vi "TestStr.vi"() -> ()   [LabVIEW 2025]
uses:
  TestStr.dll
panel:
  out "Get Char from Handle, µs":dbl format="%#.6f"
  out "byte s":u8 format="%.0x"
  out "byte h":u8 format="%.0x"
  out "Ratio":dbl
  out "Get Char from String, s":dbl format="%#_6f"
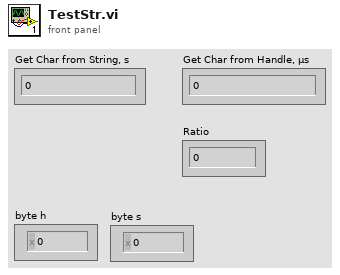
[diagram p1: front panel]
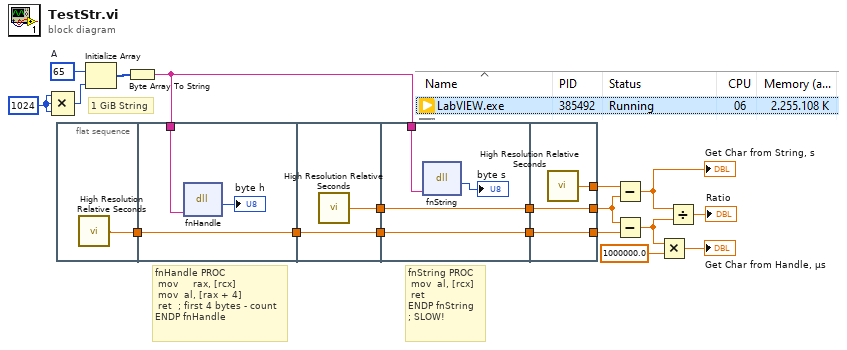
[diagram p0: block diagram]
diagram:
  w17 = 1024
  w19 = u8 65  # A
  # "1 GiB String"
  # "fnString PROC\n\tmov\t\tal, [rcx]\n\tret\nENDP fnString\n; SLOW!"
  # "fnHandle PROC\n\tmov     rax, [rcx]\n\tmov\t\tal, [rax + 4]\n\tret  ; first 4 bytes - count\nENDP fnHandle"
  n1 = Compound Arithmetic op=MULTIPLY(w17, w17, w17) -> (w16:i32)
  n2 = flat-sequence {
    tunnel: [w20] -> w6
    tunnel: w15 -> [w22]
    tunnel: [w23] -> w7
    tunnel: w6 -> [w23]
    tunnel: [w25] -> w13
    tunnel: [w24] -> w8
    tunnel: w7 -> [w24]
    tunnel: w15 -> [w27]
    tunnel: w13 -> [w29]
    tunnel: [w29] -> w12
    tunnel: [w28] -> w9
    tunnel: w8 -> [w28]
    tunnel: [w32] -> w14
    tunnel: w12 -> [w31]
    tunnel: [w31] -> w11
    tunnel: [w30] -> w10
    tunnel: w9 -> [w30]
    frame #0 {
      n3 = call <vilib>:"High Resolution Relative Seconds.vi"() -> ("relative seconds"=w20:dbl)
    }
    frame #1 {
      n4 = dll-call lib="C:/Users/Andrey/Desktop/SlowString&Search/SlowStringIssue/TestStr.dll" fn="fnHandle"("str"=w22) -> ("return type"=→"byte h":u8)  [unwired: 4 in, 2 out]
    }
    frame #2 {
      n5 = call <vilib>:"High Resolution Relative Seconds.vi"() -> ("relative seconds"=w25:dbl)
    }
    frame #3 {
      n6 = dll-call lib="C:/Users/Andrey/Desktop/SlowString&Search/SlowStringIssue/TestStr.dll" fn="fnString"("str"=w27) -> ("return type"=→"byte s":u8)  [unwired: 4 in, 2 out]
    }
    frame #4 {
      n7 = call <vilib>:"High Resolution Relative Seconds.vi"() -> ("relative seconds"=w32:dbl)
    }
  }
  n8 = Initialize Array(w19, w16) -> (w18:u8[])
  n9 = Byte Array To String(unsigned byte array=w18) -> (string=w15:string)
  n10 = Subtract(x=w14, y=w11) -> (x-y=w5:dbl)
  "Get Char from String, s" <- w5
  n11 = Subtract(x=w11, y=w10) -> (x-y=w3:dbl)
  n12 = Multiply(x=w3, y=1000000.0) -> (x*y=→"Get Char from Handle, µs":dbl)
  n13 = Divide(x=w5, y=w3) -> (x/y=→"Ratio":dbl)
